vi "Set Receive Event.vi"(8 "error in":errorcluster, 9 "Event Handle":u64, 10 "Enable":bool=TRUE, 11 "TPCANHandle in":T2=81 items=["PCAN_NONEBUS"=0, "PCAN_USBBUS1"=81, "PCAN_USBBUS2"=82, "PCAN_USBBUS3"=83, "PCAN_USBBUS4"=84, "PCAN_USBBUS5"=85, "PCAN_USBBUS6"=86, "PCAN_USBBUS7"=87, "PCAN_USBBUS8"=88, "PCAN_USBBUS9"=1289, "PCAN_USBBUS10"=1290, "PCAN_USBBUS11"=1291, "PCAN_USBBUS12"=1292, "PCAN_USBBUS13"=1293, "PCAN_USBBUS14"=1294, "PCAN_USBBUS15"=1295, "PCAN_USBBUS16"=1296]) -> (0 "error out":errorcluster, 3 "TPCANHandle out":T2=81 items=["PCAN_NONEBUS"=0, "PCAN_USBBUS1"=81, "PCAN_USBBUS2"=82, "PCAN_USBBUS3"=83, "PCAN_USBBUS4"=84, "PCAN_USBBUS5"=85, "PCAN_USBBUS6"=86, "PCAN_USBBUS7"=87, "PCAN_USBBUS8"=88, "PCAN_USBBUS9"=1289, "PCAN_USBBUS10"=1290, "PCAN_USBBUS11"=1291, "PCAN_USBBUS12"=1292, "PCAN_USBBUS13"=1293, "PCAN_USBBUS14"=1294, "PCAN_USBBUS15"=1295, "PCAN_USBBUS16"=1296], 5 "TPCANStatus":T1 items=["PCAN_ERROR_OK"=0, "PCAN_ERROR_XMTFULL"=1, "PCAN_ERROR_OVERRUN"=2, "PCAN_ERROR_BUSLIGHT"=4, "PCAN_ERROR_BUSHEAVY"=8, "PCAN_ERROR_BUSPASSIVE"=262144, "PCAN_ERROR_BUSOFF"=16, "PCAN_ERROR_QRCVEMPTY"=32, "PCAN_ERROR_QOVERRUN"=64, "PCAN_ERROR_QXMTFULL"=128, "PCAN_ERROR_REGTEST"=256, "PCAN_ERROR_NODRIVER"=512, "PCAN_ERROR_HWINUSE"=1024, "PCAN_ERROR_NETINUSE"=2048, "PCAN_ERROR_ILLHW"=5120, "PCAN_ERROR_ILLNET"=6144, "PCAN_ERROR_ILLCLIENT"=7168, "PCAN_ERROR_RESOURCE"=8192, "PCAN_ERROR_ILLPARAMTYPE"=16384, "PCAN_ERROR_ILLPARAMVAL"=32768, "PCAN_ERROR_UNKNOWN"=65536, "PCAN_ERROR_ILLDATA"=131072, "PCAN_ERROR_ILLMODE"=524288, "PCAN_ERROR_CAUTION"=33554432, "PCAN_ERROR_INITIALIZE"=67108864, "PCAN_ERROR_ILLOPERATION"=134217728])   [LabVIEW 2020, in "PCANBasic.lvlib"]
doc: "This parameter passes an event handle (Windows Event Objects) to the underlying API. This \nevent will be triggered (its state is set to “signaled”) when CAN data is placed into the receive \nqueue of a PCAN-Channel. \n\nThe PCAN-Channel must be initialized before using this parameter.\n\nEvents are normally used when an application separates processing in different execution \nthreads. In a thread, that waiting for an event to occur doesn’t affect the normal execution of \nan application. \nNote that the event is not triggered each time a message is included into the queue, but only \nwhen it states was “not signaled” and data is received. When an event is signaled, then you \nmust read the queue until emptiness and eventually reset the event (if you are using a \nmanual reset event).\n\nThe default state is disabled (0). After enabling this parameter (by configuring an event \nhandle), the PCAN-Basic API will try to signal the handle until it is disabled (by setting as \nhandle a value of 0), or the channel is disconnected (e.g., using the function \nCAN_Uninitialize).\nNote that when you need to reinitialize a PCAN-Channel, you will need to set the event again \neach time after initializing the channel, since the event will have again its default value of 0\nafter initialization. Note too that it is strongly recommended to close the handle (using \nCloseHandle) after a PCAN-Channel has been uninitialized, since the API could try to set an \ninvalid handle and this can cause undesired behavior.\n\nReturns PCAN_ERROR_ILLOPERATION on Linux as the feature is enabled by default."
uses:
  PCANBasic.lvlib
  TPCANParameter.ctl
  peak/PCANBasic64.dll
  TPCANHandle.ctl
  TPCANStatus.ctl
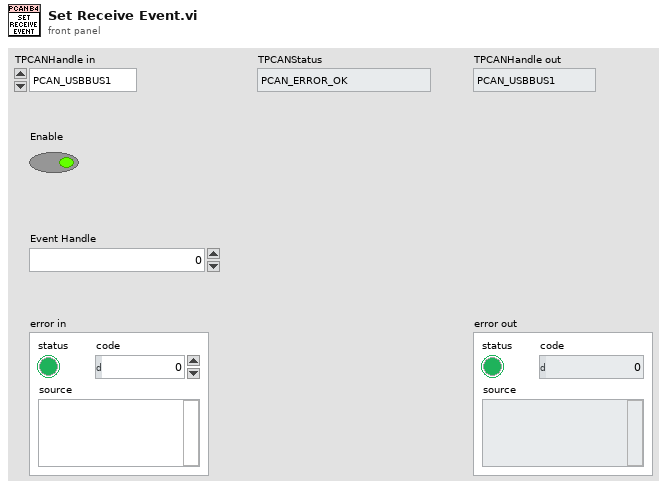
[diagram p1: front panel]
types:
  T1 = typedef "PCANBasic.lvlib/TPCANStatus.ctl" = u32
  T2 = typedef "PCANBasic.lvlib/TPCANHandle.ctl" = u16
  T3 = typedef "PCANBasic.lvlib/TPCANParameter.ctl" = enum8{"Unknown", "PCAN_DEVICE_ID", "PCAN_5VOLTS_POWER", "PCAN_RECEIVE_EVENT", "PCAN_MESSAGE_FILTER", "PCAN_API_VERSION", "PCAN_CHANNEL_VERSION", "PCAN_BUSOFF_AUTORESET", "PCAN_LISTEN_ONLY", "PCAN_LOG_LOCATION", "PCAN_LOG_STATUS", "PCAN_LOG_CONFIGURE", "PCAN_LOG_TEXT", "PCAN_CHANNEL_CONDITION", "PCAN_HARDWARE_NAME", "PCAN_RECEIVE_STATUS", "PCAN_CONTROLLER_NUMBER", "PCAN_TRACE_LOCATION", "PCAN_TRACE_STATUS", "PCAN_TRACE_SIZE", "PCAN_TRACE_CONFIGURE", "PCAN_CHANNEL_IDENTIFYING", "PCAN_CHANNEL_FEATURES", "PCAN_BITRATE_ADAPTING", "PCAN_BITRATE_INFO", "PCAN_BITRATE_INFO_FD", "PCAN_BUSSPEED_NOMINAL", "PCAN_BUSSPEED_DATA", "PCAN_IP_ADDRESS", "PCAN_LAN_SERVICE_STATUS", "PCAN_ALLOW_STATUS_FRAMES", "PCAN_ALLOW_RTR_FRAMES", "PCAN_ALLOW_ERROR_FRAMES", "PCAN_INTERFRAME_DELAY", "PCAN_ACCEPTANCE_FILTER_11BIT", "PCAN_ACCEPTANCE_FILTER_29BIT", "PCAN_IO_DIGITAL_CONFIGURATION", "PCAN_IO_DIGITAL_VALUE", "PCAN_IO_DIGITAL_SET", "PCAN_IO_DIGITAL_CLEAR", "PCAN_IO_ANALOG_VALUE", "PCAN_FIRMWARE_VERSION", "PCAN_ATTACHED_CHANNELS_COUNT", "PCAN_ATTACHED_CHANNELS", "PCAN_ALLOW_ECHO_FRAMES", "PCAN_DEVICE_PART_NUMBER", "PCAN_HARD_RESET_STATUS", "PCAN_LAN_CHANNEL_DIRECTION", "PCAN_DEVICE_GUID"}
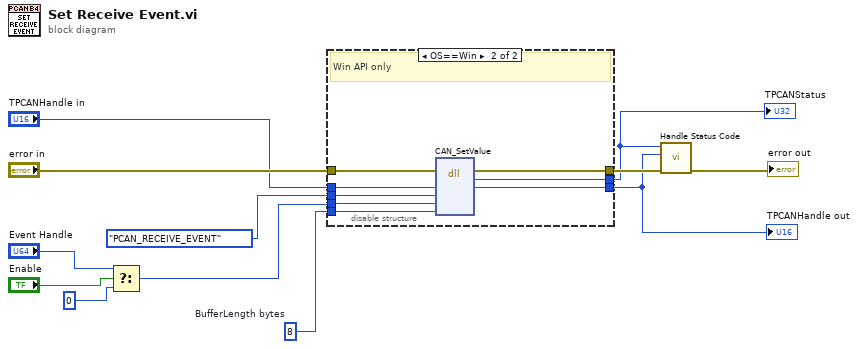
[diagram p0: block diagram]
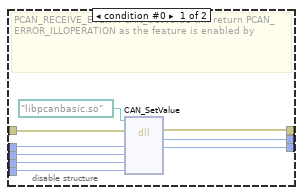
[diagram p2: hidden frame]
diagram:
  w9 = u32 8  # BufferLength bytes
  n1 = Select(t="Event Handle", s="Enable", f=u64 0) -> (s? t:f=w7:u64)
  n2 = disable-structure shown="OS==Win" {
    disable-tunnel: "error in" -> [w21 w29]
    disable-tunnel: [w20 w28] -> w11
    disable-tunnel: TPCANParameter."PCAN_RECEIVE_EVENT" ("TPCANParameter") -> [w18 w27]
    disable-tunnel: w9 -> [w16 w26]
    disable-tunnel: w7 -> [w17 w25]
    disable-tunnel: "TPCANHandle in" -> [w19 w24]
    disable-tunnel: [w15 w23] -> w2
    disable-tunnel: [w14 w22] -> w1
    frame condition #0 {
      # "PCAN_RECEIVE_EVENT: CAN_SetValue will return PCAN_ERROR_ILLOPERATION as the feature is enabled by"
      n3 = dll-call lib="libpcanbasic.so" fn="CAN_SetValue"(path in=path "libpcanbasic.so", error in=w21, "Channel"=w19, "TPCANParameter"=w18, "Buffer"=w17, "BufferLength"=w16) -> (error out=w20:errorcluster, "TPCANStatus"=w15:u32, "Channel"=w14:u16)  [unwired: 4 in, 1 out]
    }
    frame condition #1 (active) {
      # "Win API only"
      n4 = dll-call lib="D:/git/PCAN-Basic-LabVIEW/source/peak/PCANBasic*.dll" fn="CAN_SetValue"(error in=w29, "Channel"=w24, "TPCANParameter"=w27, "Buffer"=w25, "BufferLength"=w26) -> (error out=w28:errorcluster, "TPCANStatus"=w23:u32, "Channel"=w22:u16)  [unwired: 5 in, 1 out]
    }
  }
  "TPCANHandle out" <- w1
  "TPCANStatus" <- w2
  n5 = call "Handle Status Code.vi"("error in"=w11, "TPCANHandle"=w1, "TPCANStatus"=w2) -> ("error out"=→"error out":errorcluster)  [unwired: 8 in]
